vi "Select with boolean array input.vi"(1 "T string":string, 2 "F string":string, 3 "T/F":bool[](array[boolean]), 4 "Size":i32) -> (14 "String array out":string[](array[string]))   [LabVIEW 2026]
doc: "This VI returns a string array of a given size with T string and F string, depending on the boolean value at the corresponding index of T/F."
panel:
  # "This vi returns a string array of a given size with T string and F string, \ndepending on the boolean value at the corresponding index of T/F."
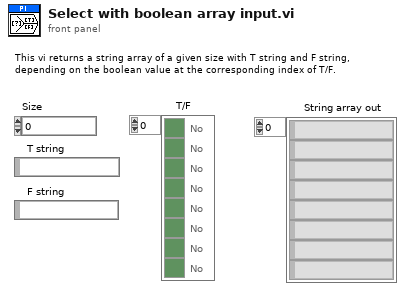
[diagram p1: front panel]
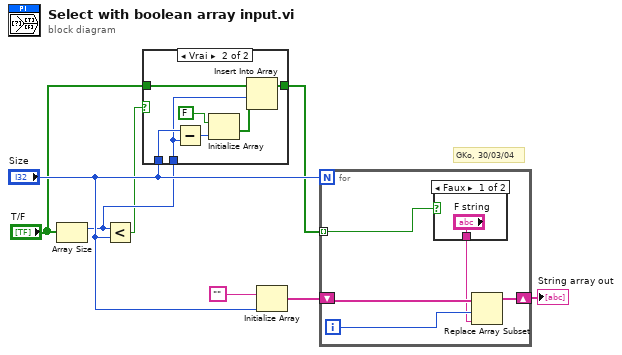
[diagram p0: block diagram]
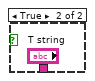
[diagram p3: hidden frame]
diagram:
  # "GKo, 30/03/04"
  n1 = Array Size(array="T/F") -> (size(s)=w4:i32)
  n2 = Less?(x=w4, y="Size") -> (x < y?=w2:bool)
  n3 = case shown="Vrai" w2 {
    tunnel: "Size" -> [_ w16]
    tunnel: w4 -> [_ w14]
    tunnel: "T/F" -> [w9 w11]
    tunnel: [w9 w10] -> w1
    frame False {
    }
    frame True {
      n4 = Subtract(x=w16, y=w14) -> (x-y=w15:i32)
      n5 = Initialize Array(FALSE ("Element Data"), w15) -> (w13:bool[])
      n6 = Insert Into Array(array=w11, index=w14, new element=w13) -> (w10:bool[])
    }
  }
  n7 = Initialize Array("" ("Element Data"), "Size") -> (w6:string[])
  n8 = for {
    N: "Size" -> [_]
    tunnel: w1 -> [w17] mode=indexing
    shift-right: [w19] -> w8
    shift-left: w6 -> [w20]
    i -> [w21]
    n9 = case shown="Faux" w17 {
      tunnel: ["F string" "T string"] -> w18
      frame False {
      }
      frame True {
      }
    }
    n10 = Replace Array Subset(array=w20, new element=w18, index=w21) -> (w19:string[])
  }
  "String array out" <- w8
